vi "区域清除.vi"(8 "偏移量":cluster{"X":i32, "Y":i32}, 9 "列":i8, 10 "行":i8, 11 "数组":u32[][](array[colorbox])) -> (3 "数组 3":u32[][](array[colorbox]))   [LabVIEW 2012]
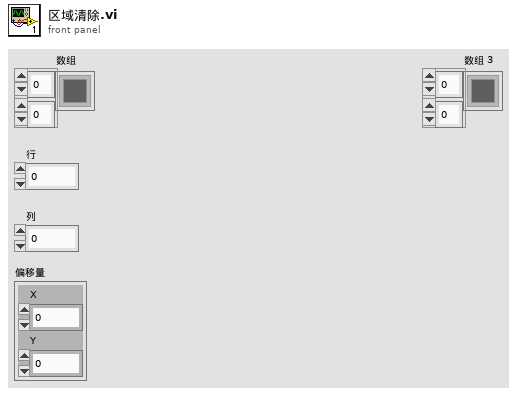
[diagram p1: front panel]
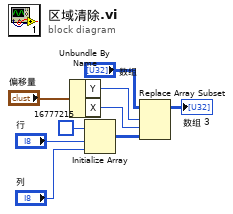
[diagram p0: block diagram]
diagram:
  n1 = Unbundle By Name("偏移量") -> ("Y"=w3:i32, "X"=w2:i32)
  n2 = Initialize Array(u32 16777215, "行", "列") -> (w4:u32[][])
  n3 = Replace Array Subset(array="数组", new element=w4, index (row)=w3, index (col)=w2) -> (→"数组 3":u32[][])
